vi "PathMainPy.vi"() -> (8 "path":path)   [LabVIEW 2023]
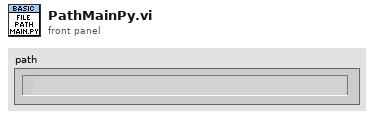
[diagram p1: front panel]
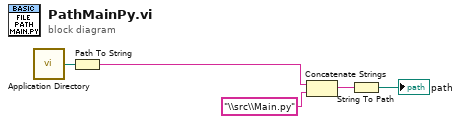
[diagram p0: block diagram]
diagram:
  n1 = call <vilib>:"Application Directory.vi"() -> ("Application Directory"=w5:path)
  n2 = Path To String(path=w5) -> (string=w1:string)
  n3 = Concatenate Strings(w1, "\\src\\Main.py" ("string")) -> (w3:string)
  n4 = String To Path(string=w3) -> (path=→"path":path)
